vi "ResonanceAnalyzer.vi"() -> ()   [LabVIEW 2015]
uses:
  <vilib>/imath/engines/lvmath2/RunTimeEngine/Managers/WorkSpace/UID Generator.vi
  <vilib>/imath/engines/lvmath2/RunTimeEngine/RangeToken/NIMS_Range.vi
  <instcachedir>/0/NIMS_Range_D919CC09935940E88F755EC1C6F49AC1.lvgen/NIMS_Range_D919CC09935940E88F755EC1C6F49AC1_000.vi
  <vilib>/imath/engines/lvmath2/RunTimeEngine/RunTimeType/NIMS_RunTimeType_From StrictType (excl LVString).vi
  <instcachedir>/0/NIMS_RunTimeType_From StrictType (excl LVString)_EB1C38A9BC5048DA9ABDA8F781E54D21.lvgen/NIMS_RunTimeType_From StrictType (excl LVString)_EB1C38A9BC5048DA9ABDA8F781E54D21_000.vi
  <vilib>/imathl/engines/lvmath/Functions/Error Handling/Create Error.vi
  <vilib>/imath/engines/lvmath2/RunTimeEngine/LocalVariableDefStatement/MC_LocalVariableDefStatement_Display.vi
  <vilib>/imath/engines/lvmath2/RunTimeEngine/BuiltInFunctions/length/NIMS_length(GV).vi
  <instcachedir>/0/NIMS_length(GV)_08A3D13377FD4E4B96F5795FBF3698FA.lvgen/NIMS_length(GV)_08A3D13377FD4E4B96F5795FBF3698FA_000.vi
  <vilib>/imath/engines/lvmath2/RunTimeEngine/RangeToken/NIMS_Range_R2 - Integer.vi
  <instcachedir>/0/NIMS_Range_R2 - Integer_396D5D4FB869421F9245109A0975AD54.lvgen/NIMS_Range_R2 - Integer_396D5D4FB869421F9245109A0975AD54_000.vi
  <vilib>/imath/engines/lvmath2/RunTimeEngine/CommandStatement/MC_CommandStatement_break.vi
  <vilib>/imath/engines/lvmath2/RunTimeEngine/VariableToken/NIMS_VariableToken_CondDefinedDefinedByReplace.vi
  <instcachedir>/0/NIMS_VariableToken_CondDefinedDefinedByReplace_D162CFFC24174562A9FEA619A91E1A56.lvgen/NIMS_VariableToken_CondDefinedDefinedByReplace_D162CFFC24174562A9FEA619A91E1A56_002.vi
  <vilib>/imath/engines/lvmath2/RunTimeEngine/IndexRead/NIMS V(S).vi
  <instcachedir>/0/NIMS V(S)_0488751826AF41519A22953C041130DC.lvgen/NIMS V(S)_0488751826AF41519A22953C041130DC_000.vi
  <vilib>/imath/engines/lvmath2/RunTimeEngine/IndexReplace/NIMS V(S)=S.vi
  <instcachedir>/0/NIMS V(S)=S_9916D32195284AEB9D40BA9A64F3B0C5.lvgen/NIMS V(S)=S_9916D32195284AEB9D40BA9A64F3B0C5_000.vi
  <vilib>/imath/engines/lvmath2/RunTimeEngine/ErrorHandling/NIMS_Create Error From Enums.vi
  <vilib>/imath/engines/lvmath2/RunTimeEngine/VariableToken/NIMS_VariableToken_CondDefined.vi
  <instcachedir>/0/NIMS_VariableToken_CondDefined_FE30D0A1BFB24F098D41DEBABFE96BE1.lvgen/NIMS_VariableToken_CondDefined_FE30D0A1BFB24F098D41DEBABFE96BE1_004.vi
  <vilib>/imath/engines/lvmath/Functions/Error Handling/MergeErrorsWrapper.vi
  <vilib>/imath/engines/lvmath2/RunTimeEngine/Managers/SymbolTable/Clear UID.vi
  <vilib>/imath/engines/lvmath2/RunTimeEngine/NodeEndStatement/NIMS_NodeEndStatement_Output.vi
  <instcachedir>/0/NIMS_NodeEndStatement_Output_53EC0D466D134D7ABD903AC30B43404B.lvgen/NIMS_NodeEndStatement_Output_53EC0D466D134D7ABD903AC30B43404B_005.vi
  <vilib>/imath/engines/lvmath2/RunTimeEngine/ErrorHandling/NIMS_Finalize Error.vi
  <vilib>/Utility/file.llb/Read Delimited Spreadsheet (DBL).vi
  <vilib>/Analysis/NI_AALBase.lvlib
  <vilib>/Analysis/NI_AALPro.lvlib
  <vilib>/imath/engines/lvmath2/RunTimeEngine/Managers/SymbolTable/NIMS_WorkSpace.lvlib
panel:
  out "Outputs":cluster{"Amplitude":dbl, "Q":dbl, "Center":dbl}={"Amplitude"=1.0040146340912846, "Q"=97.91942412365117, "Center"=609.9984195854444}
  out "XY Graph":cluster{"f":dbl[], "Best Gaussian Fit":dbl[]}[](graph)=[{"f"=[400.0, 405.0, 410.0, 415.0, 420.0, 425.0, 430.0, 435.0, 440.0, 445.0, 450.0, 455.0, 460.0, 465.0, 470.0, 475.0, 480.0, 485.0, 490.0, 495.0, 500.0, 505.0, 510.0, 515.0, 520.0, 525.0, 530.0, 535.0, 540.0, 545.0, 550.0, 555.0, 560.0, 565.0, 570.0, 575.0, 580.0, 585.0, 590.0, 595.0, 600.0, 605.0, 610.0, 615.0, 620.0, 625.0, 630.0, 635.0, 640.0, 645.0, 650.0, 655.0, 660.0, 665.0, 670.0, 675.0, 680.0, 685.0, 690.0, 695.0, 700.0, 705.0, 710.0, 715.0, 720.0, 725.0, 730.0, 735.0, 740.0, 745.0, 750.0, 755.0, 760.0, 765.0, 770.0, 775.0, 780.0, 785.0, 790.0, 795.0, 800.0], "Best Gaussian Fit"=[0.09184968652577916, 0.1611441903726241, 0.24075978321534192, 0.2185826612788643, 0.2584482245421524, 0.2578890423024309, 0.28729648681966147, 0.2569506514302669, 0.26112822759725846, 0.29630378052701617, 0.3441998608039884, 0.3077047638837772, 0.37927017014411596, 0.38681528492820805, 0.4671135191822134, 0.43894802152936485, 0.5248305609288043, 0.5393559666258845, 0.6025866777352227, 0.5735823474342469, 0.6717816836900337, 0.6739904443020098, 0.6568817852381398, 0.7076608983027229, 0.6662078745407519, 0.7314300144964753, 0.8986811479425038, 0.7455410211989606, 0.7315247756628975, 0.8297830783115695, 1.0311459756081864, 0.8142229155242108, 0.9191001300515051, 0.8691178512147916, 0.96441620821901, 0.9245596875015188, 0.9509445462031892, 0.955224611724224, 0.8836451853814041, 0.9644860842815236, 0.9810717197474432, 0.9772783873463906, 1.0461133076841111, 0.9901537331545012, 0.8896750523645492, 0.973733746053111, 0.9663455037118068, 0.9296710288829466, 0.9568679969302791, 0.8893407572167181, 1.0269707125904515, 0.8307620880714504, 0.8842900498207688, 0.8605741653812867, 0.7352794589134076, 0.7888994863992845, 0.6594619238869487, 0.7075713285054109, 0.6290305019002248, 0.5872950675033343, 0.6475585631327098, 0.5901335382647458, 0.5529570862265437, 0.5357444016275258, 0.5422656652337708, 0.46580645139006877, 0.395377975421637, 0.4277584004406064, 0.41569040709675714, 0.36958031312543016, 0.34271939898957665, 0.30487905906540846, 0.2283433923286187, 0.23474159189102203, 0.23608522049701608, 0.2372173442976574, 0.21164607504288577, 0.20801492238414837, 0.14468000486524507, 0.12884811420040213, 0.1288786263839975]}, {"f"=[400.0, 405.0, 410.0, 415.0, 420.0, 425.0, 430.0, 435.0, 440.0, 445.0, 450.0, 455.0, 460.0, 465.0, 470.0, 475.0, 480.0, 485.0, 490.0, 495.0, 500.0, 505.0, 510.0, 515.0, 520.0, 525.0, 530.0, 535.0, 540.0, 545.0, 550.0, 555.0, 560.0, 565.0, 570.0, 575.0, 580.0, 585.0, 590.0, 595.0, 600.0, 605.0, 610.0, 615.0, 620.0, 625.0, 630.0, 635.0, 640.0, 645.0, 650.0, 655.0, 660.0, 665.0, 670.0, 675.0, 680.0, 685.0, 690.0, 695.0, 700.0, 705.0, 710.0, 715.0, 720.0, 725.0, 730.0, 735.0, 740.0, 745.0, 750.0, 755.0, 760.0, 765.0, 770.0, 775.0, 780.0, 785.0, 790.0, 795.0, 800.0], "Best Gaussian Fit"=[0.10069519071641159, 0.11220224277557812, 0.12469871601450133, 0.13822610166004956, 0.15282196258348543, 0.16851909571877408, 0.1853446701735169, 0.20331935261195447, 0.22245643293698913, 0.24276096460971544, 0.2642289350745932, 0.2868464826606239, 0.31058917695992155, 0.3354213800044152, 0.3612957055333201, 0.38815259323900264, 0.4159200140751116, 0.44451332149553613, 0.4738352618631008, 0.5037761552311193, 0.5342142552787311, 0.5650162944038377, 0.5960382168886615, 0.6271260997068496, 0.6581172570023707, 0.6888415206129471, 0.7191226853156325, 0.7487801038259958, 0.7776304130750483, 0.805489370010132, 0.832173772206153, 0.8575034360159786, 0.8813032029104451, 0.9034049431265373, 0.9236495248120711, 0.9418887165678337, 0.9579869916690861, 0.9718232033061902, 0.9832921019099514, 0.9923056679943179, 0.9987942369133606, 1.0027073954305041, 1.0040146339605127, 1.0027057426804513, 0.9987909443159889, 0.9923007611873589, 0.9832856189337104, 0.9718151941124663, 0.9579775174803015, 0.9418778490978739, 0.9236373453627033, 0.9033915415753269, 0.8812886766077772, 0.8574878886100941, 0.8321573124159846, 0.8054721103661846, 0.7776124686485947, 0.7487615909664662, 0.7191037204153022, 0.6888222189168668, 0.6580977314800217, 0.6271064600002456, 0.5960185683496438, 0.5649967372311526, 0.5341948837632075, 0.5037570571149382, 0.47381651781681233, 0.44449500471419656, 0.4159021899927323, 0.3881353193584611, 0.36127903136702194, 0.33540534711935327, 0.3105738191193625, 0.2868318260534939, 0.26421499862273695, 0.24274776034256162, 0.22244396642277917, 0.20330762343455422, 0.1853336724439289, 0.16850881861077063, 0.1528123908832735]}]
  in  "?":enum32{"Simulation", "Experiment"}(tab)
  in  "Input Parameters":T1={"Q"=100.0, "Center Frequency"=600.0, "Start Frequency"=400.0, "End Frequency"=800.0, "dF"=5.0, "Noise Level "=0.05}
  in  "Fiilename":path
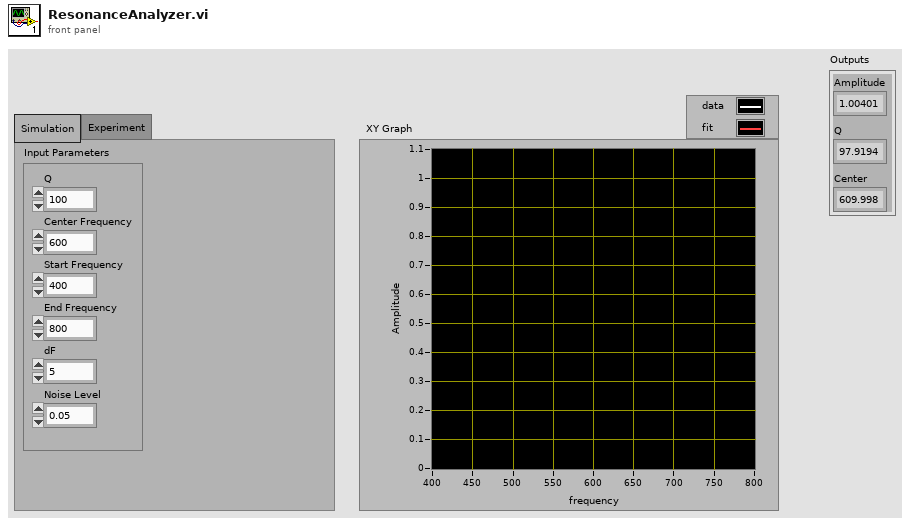
[diagram p1: front panel]
types:
  T1 = cluster{"Q":dbl, "Center Frequency":dbl, "Start Frequency":dbl, "End Frequency":dbl, "dF":dbl, "Noise Level ":dbl}
  T2 = cluster{"all rows":dbl[], "Best Gaussian Fit":dbl[]}
  T3 = cluster{"all rows":dbl[], "Best Gaussian Fit":dbl[]}[]
  T4 = cluster{"amplitude":dbl, "center":dbl, "standard deviation":dbl}
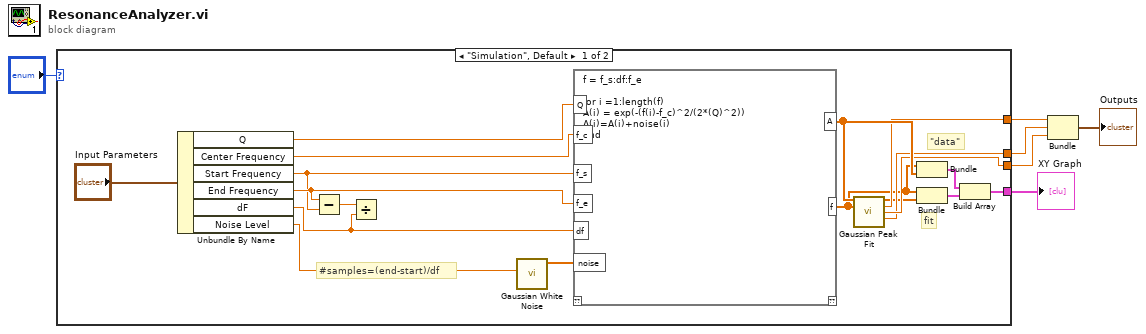
[diagram p0: block diagram]
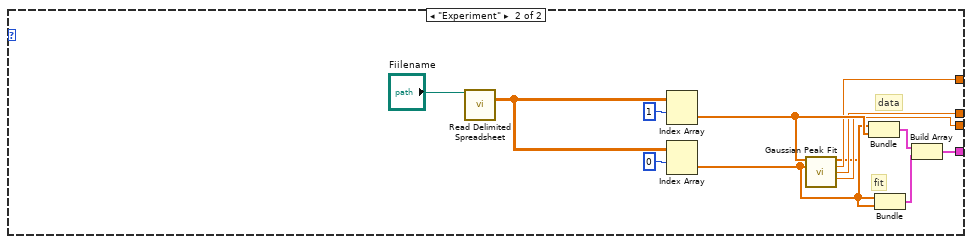
[diagram p2: hidden frame]
diagram:
  n1 = case shown="\"Simulation\", Default" "?" {
    tunnel: [w11 w229] -> w5
    tunnel: [w18 w236] -> w4
    tunnel: [w17 w234] -> w3
    tunnel: [w16 w235] -> w2
    frame "Simulation", Default {
      # "fit"
      # "\"data\""
      # "#samples=(end-start)/df"
      n2 = Unbundle By Name("Input Parameters") -> ("Q"=w23:dbl, "Center Frequency"=w22:dbl, "Start Frequency"=w9:dbl, "End Frequency"=w10:dbl, "dF"=w7:dbl, "Noise Level"=w21:dbl)
      n3 = Subtract(x=w10, y=w9) -> (x-y=w8:dbl)
      n4 = Divide(x=w8, y=w7) -> ()  [unwired: 1 out]
      n5 = call <vilib>:"Gaussian White Noise.vi"("standard deviation"=w21) -> ("Gaussian noise pattern"=w20:dbl[])  [unwired: 9 in, 1 out]
      n6 = mathscript code="f = f_s:df:f_e\n \nfor i =1:length(f)\nA(i) = exp(-(f(i)-f_c)^2/(2*(Q)^2))\nA(i)=A(i)+noise(i)\nend"("f_c"=w22, "f_e"=w10, "f_s"=w9, "df"=w7, "Q"=w23, "noise"=w20) -> ("f"=w14:dbl[], "A"=w19:dbl[])  [unwired: 1 in, 1 out]
      n7 = call <vilib>:"Gaussian Peak Fit.vi"("Y"=w19, "X"=w14) -> ("Best Gaussian Fit"=w13:dbl[], "amplitude"=w18:dbl, "center"=w17:dbl, "standard deviation"=w16:dbl)  [unwired: 7 in, 3 out]
      n8 = Bundle("f"=w14, "A"=w19) -> (w15:cluster{"f":dbl[], "A":dbl[]})  [unwired: 1 in]
      n9 = Bundle("f"=w14, "Best Gaussian Fit"=w13) -> (w12:cluster{"f":dbl[], "Best Gaussian Fit":dbl[]})  [unwired: 1 in]
      n10 = Build Array(w15, w12) -> (w11:cluster{"f":dbl[], "Best Gaussian Fit":dbl[]}[])
    }
    frame "Experiment" {
      # "fit"
      # "data"
      n11 = call-poly <vilib>:"Read Delimited Spreadsheet.vi"("file path (dialog if empty)"="Fiilename") -> ("all rows"=w240:dbl[][])  [unwired: 9 in, 5 out]
      n12 = Index Array(array=w240, index (row)=1) -> (element=w237:dbl[])  [unwired: 1 in]
      n13 = Index Array(array=w240, index (row)=0) -> (element=w232:dbl[])  [unwired: 1 in]
      n14 = call <vilib>:"Gaussian Peak Fit.vi"("Y"=w237, "X"=w232) -> ("Best Gaussian Fit"=w231:dbl[], "amplitude"=w236:dbl, "center"=w235:dbl, "standard deviation"=w234:dbl)  [unwired: 7 in, 3 out]
      n15 = Bundle("all rows"=w232, "all rows"=w237) -> (w233:cluster{"all rows":dbl[], "all rows":dbl[]})  [unwired: 1 in]
      n16 = Bundle("all rows"=w232, "Best Gaussian Fit"=w231) -> (w230:T2)  [unwired: 1 in]
      n17 = Build Array(w233, w230) -> (w229:T3)
    }
  }
  "XY Graph" <- w5
  n18 = Bundle("amplitude"=w4, "center"=w2, "standard deviation"=w3) -> (→"Outputs":T4)  [unwired: 1 in]
